vi "array.vi"() -> ()   [LabVIEW 2015]
uses:
  <vilib>/Utility/miscctls.llb/LVStringsAndValuesArrayTypeDef.ctl
panel:
  out "x .xor. y?":cluster{"Ring":u16, "Boolean":bool}[](array[cluster])
  in  "stop":bool
  in  "Multicolumn Listbox":i32(listbox)
  in  "Ring":u16(ring)
  in  "Array":cluster{"Ring":u16, "Boolean":bool}[](array[cluster]) {"Ring" items=["one", "Two"]}
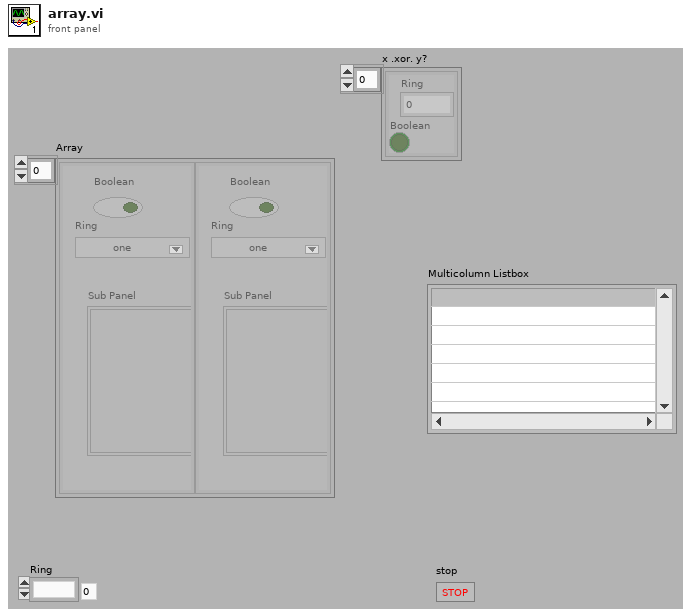
[diagram p1: front panel]
types:
  T1 = typedef "LVStringsAndValuesArrayTypeDef.ctl" = cluster{"String":string, "Value":ext}[]
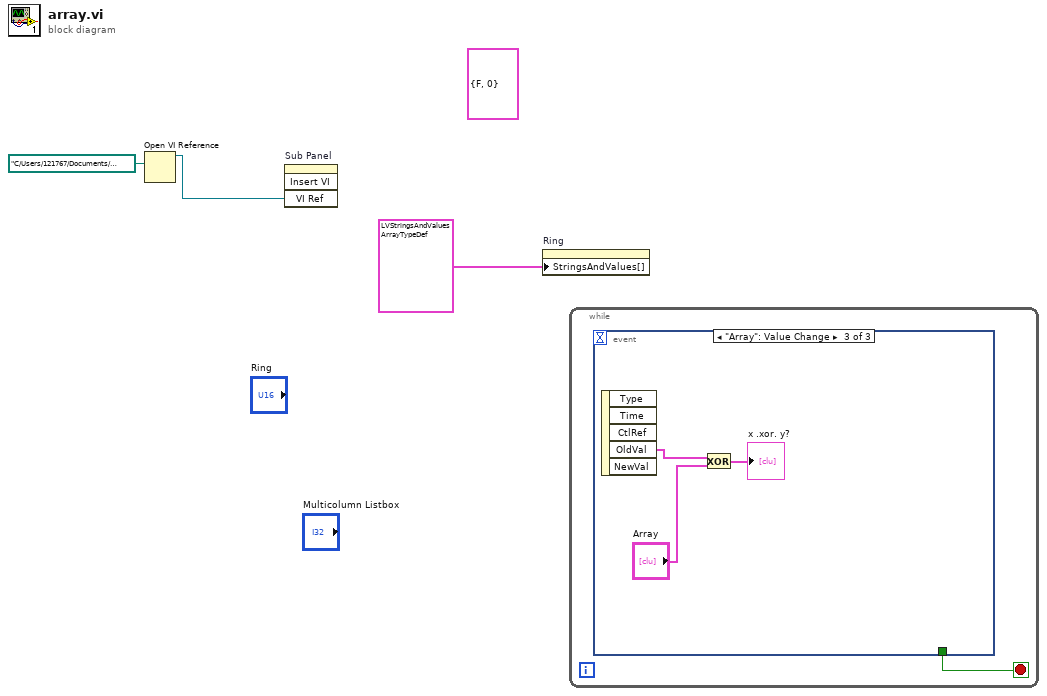
[diagram p0: block diagram]
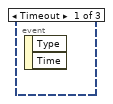
[diagram p2: hidden frame]
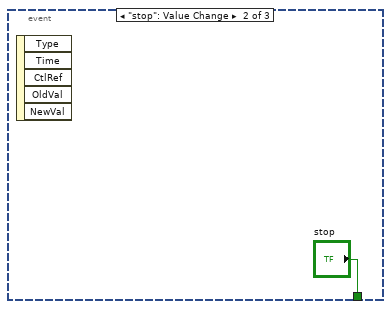
[diagram p3: hidden frame]
diagram:
  (unwired) cluster{"Boolean":bool, "Ring":u16} {"Boolean"=FALSE, "Ring"=0} ("element")
  n1 = Open VI Reference(vi path=path "C:/Users/121767/Documents/Subversion/NHMFL/Private/Fedor/Xcontrol test/2010-05/Stand alove FP.vi") -> (vi reference=w1:refnum<vi>)  [unwired: 5 in, 1 out]
  n2 = invoke on="Sub Panel" class="SubPanel" method="Insert VI"("VI Ref"=w1) -> ()  [unwired: 3 in, 4 out]
  n3 = property on="Ring" class="Ring (strict)"("StringsAndValues[]"=T1 [{"String"="one", "Value"=0.0}, {"String"="Two", "Value"=1.0}] ("Strings And Values []")) -> ()  [unwired: 2 in, 2 out]
  n4 = while {
    stop <- w4 stop-if-true
    n5 = event shown="[2] \"Array\": Value Change" {
      selector: _ -> [_ _ _]
      dyn-events: _ -> [_ _ _]
      timeout: _ -> [_ _ _]
      tunnel: [_ "stop" _] -> w4
      event Timeout {
        n6 = event-data() -> ()  [unwired: 1 in, 2 out]
      }
      event "stop": Value Change {
        n7 = event-data() -> ()  [unwired: 1 in, 5 out]
      }
      event "Array": Value Change {
        n8 = event-data() -> ("OldVal"=w8:cluster{"Ring":u16, "Boolean":bool}[])  [unwired: 1 in, 4 out]
        n9 = Exclusive Or(1:"Array", 2:w8) -> (0:→"x .xor. y?":cluster{"Ring":u16, "Boolean":bool}[])
      }
    }
  }
